vi "GetFault_TALONFX_ReverseSoftLimit.vi"(8 "error in":errorcluster, 9 "timeoutSeconds":dbl=0.05, 10 "WaitForUpdate":bool, 11 "DeviceReference":T2) -> (0 "error out":errorcluster, 3 "Output":T1)   [LabVIEW 2023]
uses:
  Users/Cory/Documents/PhoenixPro-LabVIEW-Generation/controls/DeviceReference.ctl
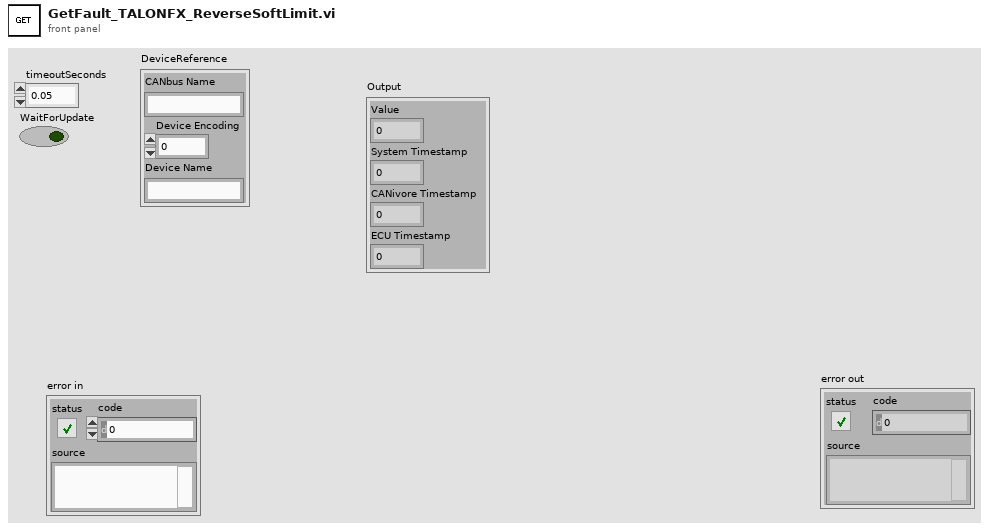
[diagram p1: front panel]
types:
  T1 = cluster{"Value":dbl, "System Timestamp":dbl, "CANivore Timestamp":dbl, "ECU Timestamp":dbl}
  T2 = typedef "DeviceReference.ctl" = cluster{"CANbus Name":string, "Device Encoding":u32, "Device Name":string}
  T3 = cluster{"OutValue":dbl, "Units":cluster{"Numeric":u8, "Numeric 2":u8, "Numeric 3":u8, "Numeric 4":u8, "Numeric 5":u8, "Numeric 6":u8, "Numeric 7":u8, "Numeric 8":u8, "Numeric 9":u8, "Numeric 10":u8}, "swTimestampSeconds":dbl, "hwTimestampSeconds":dbl, "ecuTimestampSeconds":dbl, "error":i32}
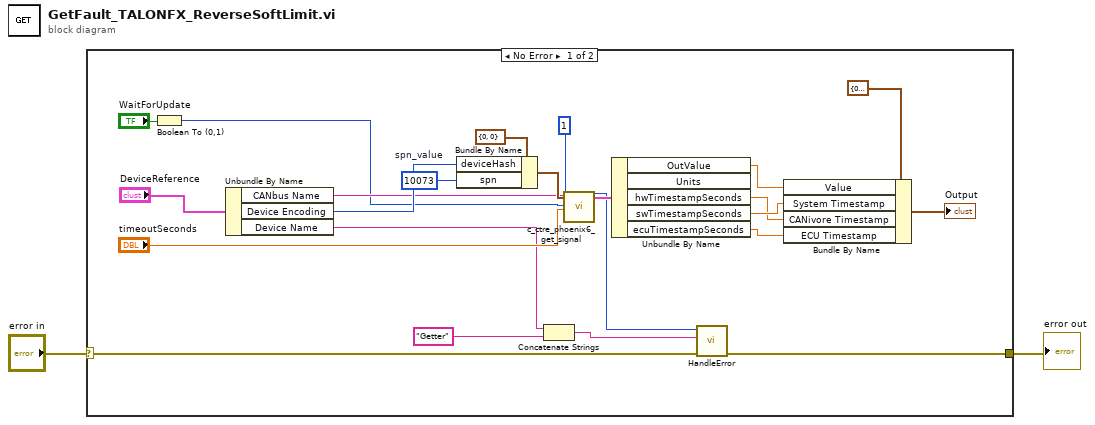
[diagram p0: block diagram]
diagram:
  n1 = case shown="No Error" "error in" {
    selector: "error in" -> [w7 w26]
    tunnel: [w6 w26] -> w1
    frame No Error {
      w18 = u32 10073  # spn_value
      n2 = Boolean To (0,1)(Boolean="WaitForUpdate") -> (0, 1=w10:i16)
      n3 = Unbundle By Name("DeviceReference") -> ("CANbus Name"=w11:string, "Device Encoding"=w19:u32, "Device Name"=w4:string)
      n4 = Bundle By Name(cluster=cluster{"deviceHash":u32, "spn":u32} {"deviceHash"=0, "spn"=0} ("Cluster"), "deviceHash"=w19, "spn"=w18) -> (w20:cluster{"deviceHash":u32, "spn":u32})
      n5 = Concatenate Strings(w4, "Getter" ("origin")) -> (w3:string)
      n6 = call <vilib>:"c_ctre_phoenix6_get_signal.vi"("Numeric 2"=u32 1 ("num_signals"), "Cluster"=w20, "String 2"=w11, "Numeric 3"=w10, "Numeric 4"="timeoutSeconds") -> ("Numeric"=w8:i32, "Cluster 2"=w16:T3)  [unwired: 20 in, 1 out]
      n7 = Unbundle By Name(w16) -> ("OutValue"=w15:dbl, "hwTimestampSeconds"=w13:dbl, "swTimestampSeconds"=w14:dbl, "ecuTimestampSeconds"=w12:dbl)  [unwired: 1 out]
      n8 = call "HandleError.vi"("error in"=w7, "origin"=w3, "Status"=w8) -> ("error out"=w6:errorcluster)  [unwired: 8 in]
      n9 = Bundle By Name(cluster=T1 {"Value"=0.0, "System Timestamp"=0.0, "CANivore Timestamp"=0.0, "ECU Timestamp"=0.0} ("Output 2"), "Value"=w15, "System Timestamp"=w14, "CANivore Timestamp"=w13, "ECU Timestamp"=w12) -> (→"Output":T1)
    }
    frame Error {
    }
  }
  "error out" <- w1
